vi "terminate.vi"(8 "error in (no error)":errorcluster, 11 "GenericPlugin in":refnum<class "TrajectoryMG100122GenericFPGA.lvclass">) -> (0 "error out":errorcluster, 3 "GenericPlugin out":refnum<class "TrajectoryMG100122GenericFPGA.lvclass">)   [LabVIEW 2010, in "TrajectoryMG100122GenericFPGA.lvclass"]
doc: "The dynamic dispatch version of this VI terminates the plug-in object by releasing all of its resources."
uses:
  TrajectoryMG100122GenericFPGA.lvclass
  FPGAWrapper/GenericFPGAWrapper/GenericFPGAWrapper/GenericFPGAWrapper.lvclass
  GenericTrajectory/GenericTrajectory/GenericTrajectory.lvclass
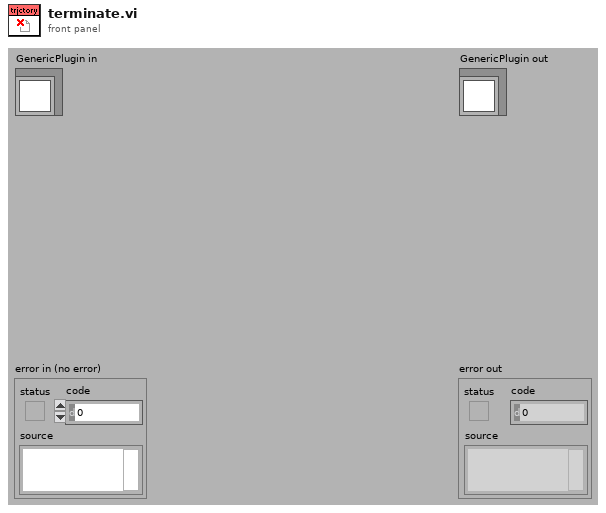
[diagram p1: front panel]
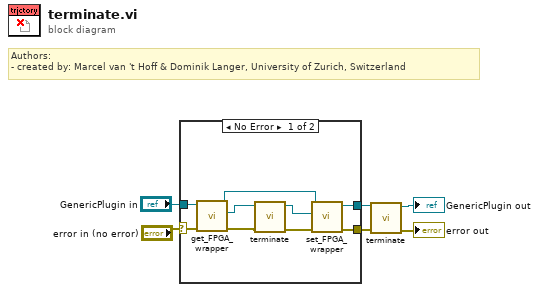
[diagram p0: block diagram]
diagram:
  # "Authors: \n- created by: Marcel van 't Hoff & Dominik Langer, University of Zurich, Switzerland"
  n1 = case shown="No Error" "error in (no error)" {
    selector: "error in (no error)" -> [w14 w16]
    tunnel: "GenericPlugin in" -> [w10 w17]
    tunnel: [w8 w16] -> w2
    tunnel: [w7 w17] -> w1
    frame No Error {
      n2 = call-dynamic "get_FPGA_wrapper.vi"("error in (no error)"=w14, "TrajectoryMG100122GenericFPGA in"=w10) -> ("error out"=w13:errorcluster, "GenericFPGAWrapper.lvclass"=w11:refnum<class "GenericFPGAWrapper.lvclass">, "TrajectoryMG100122GenericFPGA out"=w15:refnum<class "TrajectoryMG100122GenericFPGA.lvclass">)  [unwired: 7 in]
      n3 = call-dynamic "terminate.vi"("error in (no error)"=w13, "GenericPlugin in"=w11) -> ("error out"=w12:errorcluster, "GenericPlugin out"=w9:refnum<class "GenericFPGAWrapper.lvclass">)  [unwired: 8 in]
      n4 = call-dynamic "set_FPGA_wrapper.vi"("error in (no error)"=w12, "GenericFPGAWrapper.lvclass"=w9, "TrajectoryMG100122GenericFPGA in"=w15) -> ("error out"=w8:errorcluster, "TrajectoryMG100122GenericFPGA out"=w7:refnum<class "TrajectoryMG100122GenericFPGA.lvclass">)  [unwired: 7 in]
    }
    frame Error {
    }
  }
  n5 = call-parent "terminate.vi"("error in (no error)"=w2, "GenericPlugin in"=w1) -> ("error out"=→"error out":errorcluster, "GenericPlugin out"=→"GenericPlugin out":refnum<class "TrajectoryMG100122GenericFPGA.lvclass">)  [unwired: 8 in]
